vi "7442.vi"(0 "D":bool, 5 "C":bool, 7 "B":bool, 9 "A":bool) -> (1 "0":bool, 2 "1":bool, 3 "2":bool, 4 "3":bool, 6 "4":bool, 8 "5":bool, 10 "6":bool, 13 "9":bool, 14 "8":bool, 15 "7":bool)   [LabVIEW 2012]
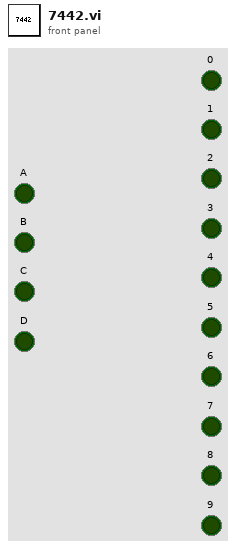
[diagram p1: front panel]
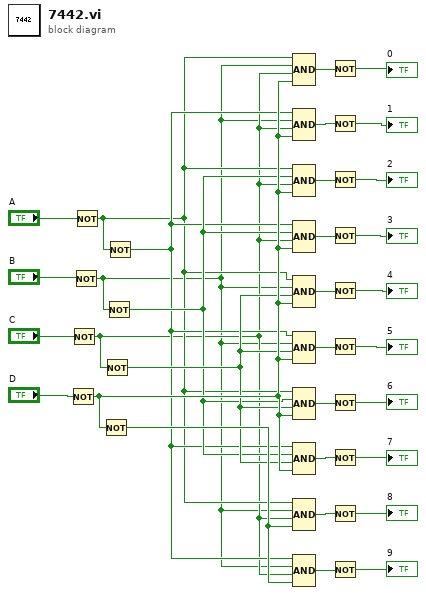
[diagram p0: block diagram]
diagram:
  n1 = Not(x="D") -> (.not. x?=w8:bool)
  n2 = Not(x="C") -> (.not. x?=w2:bool)
  n3 = Not(x="B") -> (.not. x?=w1:bool)
  n4 = Not(x="A") -> (.not. x?=w3:bool)
  n5 = Not(x=w8) -> (.not. x?=w7:bool)
  n6 = Not(x=w2) -> (.not. x?=w6:bool)
  n7 = Not(x=w1) -> (.not. x?=w5:bool)
  n8 = Not(x=w3) -> (.not. x?=w4:bool)
  n9 = Compound Arithmetic op=AND(w3, w1, w2, w8) -> (w32:bool)
  n10 = Compound Arithmetic op=AND(w4, w1, w2, w8) -> (w31:bool)
  n11 = Compound Arithmetic op=AND(w3, w5, w2, w8) -> (w29:bool)
  n12 = Compound Arithmetic op=AND(w4, w5, w2, w8) -> (w30:bool)
  n13 = Compound Arithmetic op=AND(w3, w1, w6, w8) -> (w28:bool)
  n14 = Compound Arithmetic op=AND(w4, w1, w6, w8) -> (w23:bool)
  n15 = Compound Arithmetic op=AND(w3, w5, w6, w8) -> (w24:bool)
  n16 = Compound Arithmetic op=AND(w4, w5, w6, w8) -> (w26:bool)
  n17 = Compound Arithmetic op=AND(w3, w1, w2, w7) -> (w25:bool)
  n18 = Compound Arithmetic op=AND(w4, w1, w2, w7) -> (w27:bool)
  n19 = Not(x=w32) -> (.not. x?=→"0":bool)
  n20 = Not(x=w31) -> (.not. x?=→"1":bool)
  n21 = Not(x=w29) -> (.not. x?=→"2":bool)
  n22 = Not(x=w30) -> (.not. x?=→"3":bool)
  n23 = Not(x=w28) -> (.not. x?=→"4":bool)
  n24 = Not(x=w23) -> (.not. x?=→"5":bool)
  n25 = Not(x=w24) -> (.not. x?=→"6":bool)
  n26 = Not(x=w26) -> (.not. x?=→"7":bool)
  n27 = Not(x=w25) -> (.not. x?=→"8":bool)
  n28 = Not(x=w27) -> (.not. x?=→"9":bool)
